vi "Subvi temp.vi"(0 "Temperature F":dbl, 10 "Boolean":bool) -> (4 "Numeric":dbl)   [LabVIEW 2018]
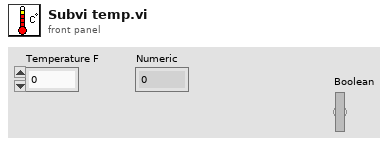
[diagram p1: front panel]
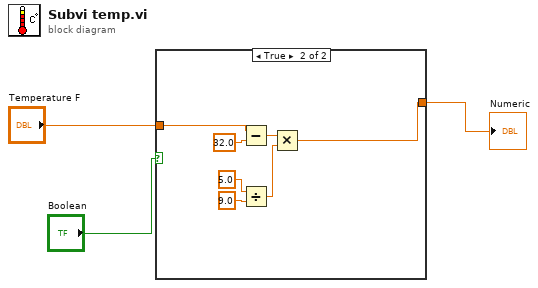
[diagram p0: block diagram]
diagram:
  n1 = case shown="True" "Boolean" {
    tunnel: "Temperature F" -> [w4 w6]
    tunnel: [w4 w5] -> w2
    frame False {
    }
    frame True {
      n2 = Subtract(x=w6, y=32.0) -> (x-y=w10:dbl)
      n3 = Divide(x=5.0, y=9.0) -> (x/y=w11:dbl)
      n4 = Multiply(x=w10, y=w11) -> (x*y=w5:dbl)
    }
  }
  "Numeric" <- w2
